vi "Get FeedManager Pkg Path.vi"(11 "error in (no error)":errorcluster) -> (4 "Pkg Path":path, 15 "error out":errorcluster)   [LabVIEW 2021, in "Measurement Builder.lvlib"]
uses:
  Measurement Builder.lvlib
  Path Functions/Path Functions.lvlib
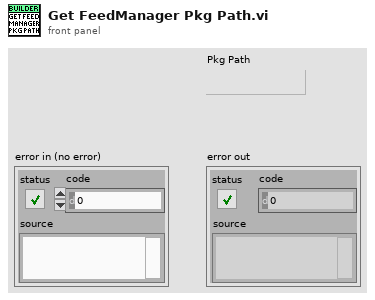
[diagram p1: front panel]
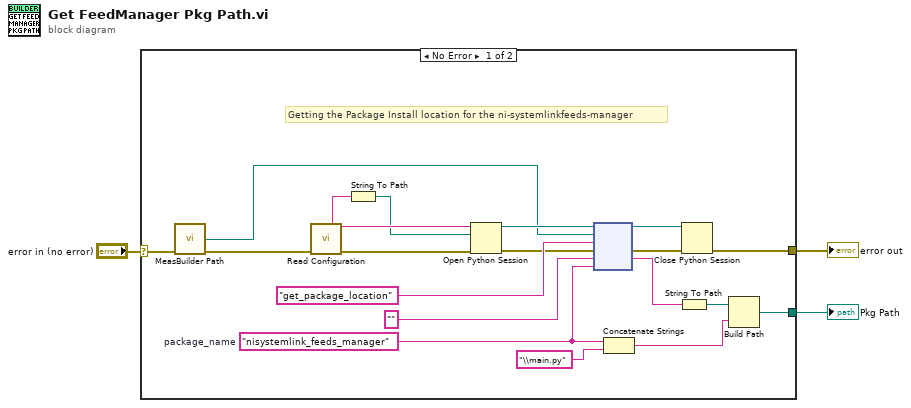
[diagram p0: block diagram]
diagram:
  n1 = case shown="No Error" "error in (no error)" {
    selector: "error in (no error)" -> [w16 w24]
    tunnel: [w10 w24] -> w2
    tunnel: [w4 _] -> w1
    frame No Error {
      w7 = "nisystemlink_feeds_manager"  # package_name
      # "Getting the Package Install location for the ni-systemlinkfeeds-manager"
      n2 = call "MeasBuilder Path.vi"("error in (no error)"=w16) -> ("Python File"=w17:path, "error out"=w15:errorcluster)  [unwired: 11 in, 2 out]
      n3 = call "Read Configuration.vi"("error in (no error)"=w15) -> ("PythonPath"=w12:string, "PythonVersion"=w14:string, "error out"=w13:errorcluster)  [unwired: 9 in, 3 out]
      n4 = String To Path(string=w12) -> (path=w11:path)
      n5 = Open Python Session(python version=w14, python path=w11, 3:w13) -> (session out=w18:refnum<k35>, error out=w19:errorcluster)
      n6 = node(w18, w17, "get_package_location" ("Python version"), w19, "", w7) -> (w23:refnum<k35>, w22:errorcluster, w9:string)  [unwired: 1 in, 2 out]
      n7 = Concatenate Strings(w7, "\\main.py" ("string")) -> (w5:string)
      n8 = String To Path(string=w9) -> (path=w8:path)
      n9 = Close Python Session(session in=w23, error in=w22) -> (11:w10:errorcluster)
      n10 = Build Path(base path=w8, name or relative path=w5) -> (appended path=w4:path)
    }
    frame Error {
    }
  }
  "error out" <- w2
  "Pkg Path" <- w1
